vi "命令读写.vi"(0 "连接ID":refnum<k5>, 2 "输入簇":T1) -> (14 "连接ID输出":refnum<k5>, 15 "输出簇":T1)   [LabVIEW 2019]
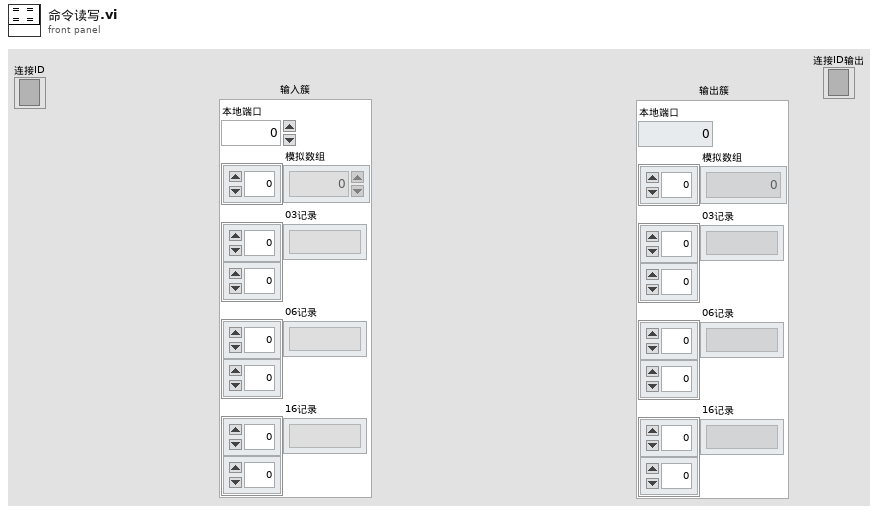
[diagram p1: front panel]
types:
  T1 = cluster{"本地端口":u16, "模拟数组":u16[], "03记录":string[][], "06记录":string[][], "16记录":string[][]}
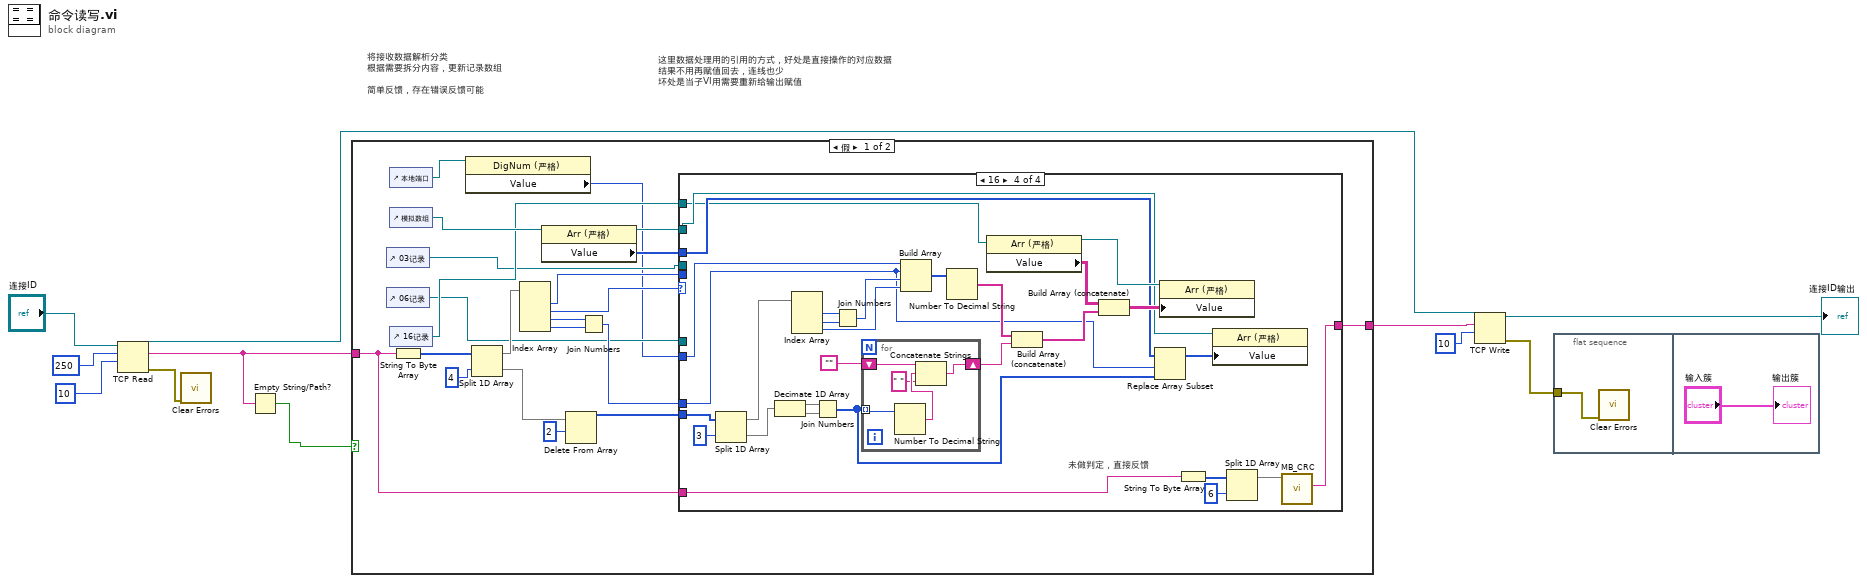
[diagram p0: block diagram]
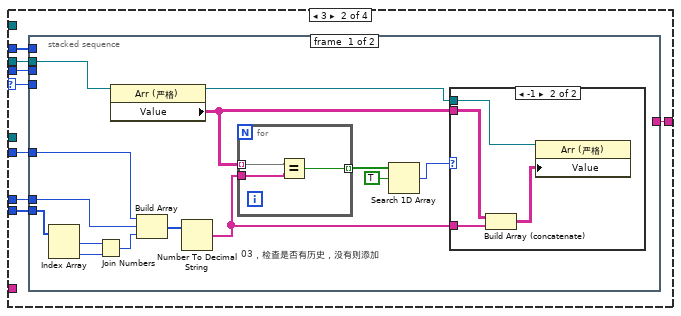
[diagram p3: hidden frame]
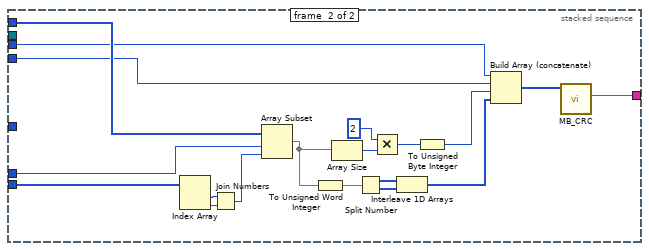
[diagram p5: hidden frame]
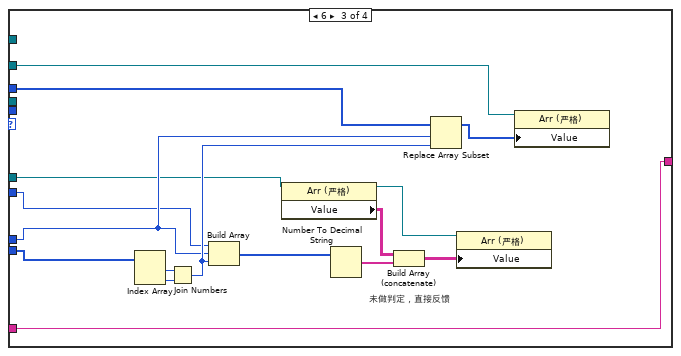
[diagram p6: hidden frame]
diagram:
  # "这里数据处理用的引用的方式，好处是直接操作的对应数据\n结果不用再赋值回去，连线也少\n坏处是当子VI用需要重新给输出赋值"
  # "将接收数据解析分类\n根据需要拆分内容，更新记录数组\n\n简单反馈，存在错误反馈可能"
  n1 = TCP Read(connection ID="连接ID", bytes to read=250 ("读取的字节"), 9:10 ("超时毫秒(25000)")) -> (connection ID out=w5:refnum<k5>, data out=w8:string, error out=w1:errorcluster)  [unwired: 2 in]
  n2 = call <vilib>:"Clear Errors.vi"("error in (no error)"=w1) -> ()  [unwired: 5 in, 2 out]
  n3 = Empty String/Path?(string/path=w8) -> (empty?=w2:bool)
  n4 = case shown="假" w2 {
    tunnel: w8 -> [w32 w132]
    tunnel: [w30 w132] -> w7
    frame False {
      n5 = control-ref of="03记录"() -> (w14:refnum<vi>)
      n6 = control-ref of="06记录"() -> (w15:refnum<vi>)
      n7 = control-ref of="本地端口"() -> (w13:refnum<vi>)
      n8 = control-ref of="模拟数组"() -> (w17:refnum<vi>)
      n9 = control-ref of="16记录"() -> (w16:refnum<vi>)
      n10 = String To Byte Array(string=w32) -> (unsigned byte array=w26:u8[])
      n11 = property class="DigNum (严格)"(reference=w13) -> ("Value"=w12:u16)  [unwired: 1 in, 2 out]
      n12 = Split 1D Array(array=w26, index=4 ("索引")) -> (first subarray=w27:u8[], second subarray=w20:u8[])
      n13 = Index Array(array=w27) -> (element #1=w31:u8, element #2=w23:u8, element #3=w28:u8, element #4=w29:u8)  [unwired: 4 in]
      n14 = property on="属性节点" class="Arr (严格)"(reference=w17) -> (reference out=w18:refnum<vi>, "Value"=w19:u16[])  [unwired: 1 in, 1 out]
      n15 = Delete From Array(array=w20, length=2 ("长度")) -> (array with subset deleted=w22:u8[])  [unwired: 1 in, 1 out]
      n16 = Join Numbers(hi=w28, lo=w29) -> ((hi.lo)=w21:u16)
      n17 = case shown="16" w23 {
        selector: w23 -> [_ w35 _ _]
        tunnel: w22 -> [_ w39 w84 w104]
        tunnel: w21 -> [_ w40 w83 w102]
        tunnel: w19 -> [_ w38 w87 w98]
        tunnel: [_ w37 w96 w122] -> w30
        tunnel: w32 -> [_ _ w96 w123]
        tunnel: w31 -> [_ w36 _ _]
        tunnel: w18 -> [_ _ w86 w99]
        tunnel: w12 -> [_ w34 w82 w103]
        tunnel: w14 -> [_ w33 _ _]
        tunnel: w15 -> [_ _ w81 _]
        tunnel: w16 -> [_ _ _ w97]
        frame 0, Default {
        }
        frame 3 {
          n18 = stacked-sequence {
            tunnel: w40 -> [w45 w80]
            tunnel: w39 -> [w43 w79]
            tunnel: w38 -> [_ w78]
            tunnel: [_ w77] -> w37
            tunnel: w36 -> [_ w76]
            tunnel: w35 -> [_ w75]
            tunnel: w34 -> [w42 _]
            tunnel: w33 -> [w41 _]
            frame #0 {
              # "03，检查是否有历史，没有则添加"
              n19 = Index Array(array=w43) -> (element #1=w53:u8, element #2=w52:u8)  [unwired: 2 in]
              n20 = Join Numbers(hi=w53, lo=w52) -> ((hi.lo)=w54:u16)
              n21 = property on="属性节点" class="Arr (严格)"(reference=w41) -> (reference out=w44:refnum<vi>, "Value"=w51:string[][])  [unwired: 1 in, 1 out]
              n22 = Build Array(w42, w45, w54) -> (w46:u16[])
              n23 = Number To Decimal String(number=w46) -> (decimal integer string=w50:string[])  [unwired: 1 in]
              n24 = for {
                tunnel: w50 -> [w60]
                tunnel: w51 -> [w61] mode=indexing
                tunnel: [w59] -> w47 mode=indexing
                n25 = Equal?(x=w61, y=w60) -> (x = y?=w59:bool)
              }
              n26 = Search 1D Array(1D array=w47, element=TRUE ("元素")) -> (index of element=w49:i32)  [unwired: 1 in]
              n27 = case shown="-1" w49 {
                tunnel: w50 -> [_ w58]
                tunnel: w51 -> [_ w57]
                tunnel: w44 -> [_ w55]
                frame 0, Default {
                }
                frame -1 {
                  n28 = Build Array (concatenate)(w57, w58) -> (w56:string[][])
                  n29 = property on="属性节点" class="Arr (严格)"(reference=w55, "Value"=w56) -> ()  [unwired: 1 in, 2 out]
                }
              }
            }
            frame #1 {
              n30 = Index Array(array=w79) -> (element #1=w73:u8, element #2=w74:u8)  [unwired: 2 in]
              n31 = Join Numbers(hi=w73, lo=w74) -> ((hi.lo)=w72:u16)
              n32 = Array Subset(array=w78, index=w80, length=w72) -> (w66:u16[])
              n33 = To Unsigned Word Integer(number=w66) -> (unsigned 16bit integer=w65:u16[])
              n34 = Array Size(array=w66) -> (size(s)=w71:i32)
              n35 = Split Number(x=w65) -> (hi(x)=w64:u8[], lo(x)=w63:u8[])
              n36 = Multiply(x=2, y=w71) -> (x*y=w69:i32)
              n37 = Interleave 1D Arrays(w64, w63) -> (w62:u8[])
              n38 = To Unsigned Byte Integer(number=w69) -> (unsigned 8bit integer=w68:u8)
              n39 = Build Array (concatenate)(w76, w75, w68, w62) -> (w67:u8[])
              n40 = call "MB_CRC.vi"("无校验U8数组"=w67) -> ("下发报文"=w77:string)  [unwired: 6 in, 1 out]
            }
          }
        }
        frame 6 {
          # "未做判定，直接反馈"
          n41 = Index Array(array=w84) -> (element #1=w92:u8, element #2=w91:u8)  [unwired: 2 in]
          n42 = Join Numbers(hi=w92, lo=w91) -> ((hi.lo)=w95:u16)
          n43 = Build Array(w82, w83, w95) -> (w89:u16[])
          n44 = property on="属性节点" class="Arr (严格)"(reference=w81) -> (reference out=w88:refnum<vi>, "Value"=w93:string[][])  [unwired: 1 in, 1 out]
          n45 = Number To Decimal String(number=w89) -> (decimal integer string=w90:string[])  [unwired: 1 in]
          n46 = Build Array (concatenate)(w93, w90) -> (w94:string[][])
          n47 = Replace Array Subset(array=w87, new element=w95, index=w83) -> (w85:u16[])
          n48 = property on="属性节点" class="Arr (严格)"(reference=w88, "Value"=w94) -> ()  [unwired: 1 in, 2 out]
          n49 = property on="属性节点" class="Arr (严格)"(reference=w86, "Value"=w85) -> ()  [unwired: 1 in, 2 out]
        }
        frame 16 {
          # "未做判定，直接反馈"
          n50 = Split 1D Array(array=w104, index=3 ("索引")) -> (first subarray=w106:u8[], second subarray=w112:u8[])
          n51 = Decimate 1D Array(w112) -> (w113:u8[], w114:u8[])
          n52 = Index Array(array=w106) -> (element #1=w107:u8, element #2=w108:u8, element #3=w110:u8)  [unwired: 3 in]
          n53 = Join Numbers(hi=w113, lo=w114) -> ((hi.lo)=w121:u16[])
          n54 = Join Numbers(hi=w107, lo=w108) -> ((hi.lo)=w109:u16)
          n55 = for {
            tunnel: w121 -> [w131] mode=indexing
            shift-right: [w128] -> w117
            shift-left: "" -> [w127]
            n56 = Number To Decimal String(number=w131) -> (decimal integer string=w130:string)  [unwired: 1 in]
            n57 = Concatenate Strings(w127, w130, " " ("字符串")) -> (w128:string)
          }
          n58 = Build Array(w103, w102, w109, w110) -> (w111:u16[])
          n59 = Number To Decimal String(number=w111) -> (decimal integer string=w116:string[])  [unwired: 1 in]
          n60 = property on="属性节点" class="Arr (严格)"(reference=w97) -> (reference out=w101:refnum<vi>, "Value"=w118:string[][])  [unwired: 1 in, 1 out]
          n61 = Build Array (concatenate)(w116, w117) -> (w119:string[])
          n62 = Build Array (concatenate)(w118, w119) -> (w120:string[][])
          n63 = Replace Array Subset(array=w98, new element=w121, index=w102) -> (w100:u16[])
          n64 = property on="属性节点" class="Arr (严格)"(reference=w101, "Value"=w120) -> ()  [unwired: 1 in, 2 out]
          n65 = String To Byte Array(string=w123) -> (unsigned byte array=w126:u8[])
          n66 = property on="属性节点" class="Arr (严格)"(reference=w99, "Value"=w100) -> ()  [unwired: 1 in, 2 out]
          n67 = Split 1D Array(array=w126, index=6 ("索引")) -> (first subarray=w124:u8[])  [unwired: 1 out]
          n68 = call "MB_CRC.vi"("无校验U8数组"=w124) -> ("下发报文"=w122:string)  [unwired: 6 in, 1 out]
        }
      }
    }
    frame True {
    }
  }
  n69 = TCP Write(connection ID=w5, data in=w7, 9:10 ("超时毫秒(25000)")) -> (connection ID out=→"连接ID输出":refnum<k5>, error out=w4:errorcluster)  [unwired: 1 in, 1 out]
  n70 = flat-sequence {
    tunnel: w4 -> [w133]
    frame #0 {
      n71 = call <vilib>:"Clear Errors.vi"("error in (no error)"=w133) -> ()  [unwired: 5 in, 2 out]
    }
    frame #1 {
      "输出簇" <- "输入簇"
    }
  }
